vi "Noise (G3)-Create (Inverse Filtered).vi"(0 "Noise In":T6={"Properties"={"InvFilt"=TRUE, "Aweight"=FALSE, "Seed"=0, "Tokens"=0, "Brickwall"=FALSE}, "Data"={"TokenNum"=0}}, 5 "Level In":T4={"Level"=65.0, "Units"=enum."dB SPL", "Max"=129.40374449454038, "Data"={"Multiplier"=0.0, "Cal File"=path "C:/Data/Calibrations/InsertRight.calib", "Cal"={"Freq (Hz)"=array[999 elements], "Mag (dB SPL)"=array[999 elements], "Phase (deg)"=array[999 elements]}, "audiogram"=path "C:/Data/XYZ DATA/XYZ999/Right.txt"}}, 7 "Filter In":T1={"Type"=enum."Bandpass", "CF (kHz)"=3.0, "BW (kHz)"=1.0, "Cascade"=FALSE, "Quadrature"=FALSE, "Scale Factor"=0.618300269961, "Stages"=[{"IIR Filter"={"filter structure"=enum."IIR 4th Order", "Reverse Coefficients"=[-0.201940179927, 0.9304964170487, -0.1627584962201, 0.7169277799719, -0.188771055144, 0.7375967101194, -0.1003225284339, 0.3609942594263, -0.1818754527879, 0.63659078182, -0.06762987697315, 0.1746207484038, -0.1788768489915, 0.5926676052203, -0.05341323516015, 0.09357484569324], "Forward Coefficients"=[0.1997628457009, 0.0, -0.3995256914017, 0.0, 0.1997628457009, 0.1583503333203, 0.0, -0.3167006666407, 0.0, 0.1583503333203, 0.1366659600116, 0.0, -0.2733319200231, 0.0, 0.1366659600116, 0.1272363495488, 0.0, -0.2544726990976, 0.0, 0.1272363495488]}, "State"=[]}], "Class"=enum."Butterworth", "Order"=8, "BWUnits"=enum."Linear"} {"Stages"."IIR Filter"."Forward Coefficients" format="%.4f"; "Stages"."IIR Filter"."Reverse Coefficients" format="%.4f"}, 9 "Fs (Hz)":dbl=50000.0, 11 "error in (no error)":errorcluster, 12 "Token length (s)":dbl=7.146) -> (4 "Noise Out":T6={"Properties"={"InvFilt"=TRUE, "Aweight"=FALSE, "Seed"=0, "Tokens"=0, "Brickwall"=FALSE}, "Data"={"TokenNum"=0}}, 6 "Level Out":T4={"Level"=65.0, "Units"=enum."dB SPL", "Max"=129.02741664769067, "Data"={"Multiplier"=0.0, "Cal File"=path "C:/Data/Calibrations/InsertRight.calib", "Cal"={"Freq (Hz)"=array[999 elements], "Mag (dB SPL)"=array[999 elements], "Phase (deg)"=array[999 elements]}, "audiogram"=path "C:/Data/XYZ DATA/XYZ999/Right.txt"}}, 8 "Filter Out":T1={"Type"=enum."Bandpass", "CF (kHz)"=3.0, "BW (kHz)"=1.0, "Cascade"=FALSE, "Quadrature"=FALSE, "Scale Factor"=0.618300269961, "Stages"=[{"IIR Filter"={"filter structure"=enum."IIR 4th Order", "Reverse Coefficients"=[-0.201940179927, 0.9304964170487, -0.1627584962201, 0.7169277799719, -0.188771055144, 0.7375967101194, -0.1003225284339, 0.3609942594263, -0.1818754527879, 0.63659078182, -0.06762987697315, 0.1746207484038, -0.1788768489915, 0.5926676052203, -0.05341323516015, 0.09357484569324], "Forward Coefficients"=[0.1997628457009, 0.0, -0.3995256914017, 0.0, 0.1997628457009, 0.1583503333203, 0.0, -0.3167006666407, 0.0, 0.1583503333203, 0.1366659600116, 0.0, -0.2733319200231, 0.0, 0.1366659600116, 0.1272363495488, 0.0, -0.2544726990976, 0.0, 0.1272363495488]}, "State"=[]}], "Class"=enum."Butterworth", "Order"=8, "BWUnits"=enum."Linear"} {"Stages"."IIR Filter"."Forward Coefficients" format="%.4f"; "Stages"."IIR Filter"."Reverse Coefficients" format="%.4f"}, 10 "InvFilter Noise":dbl[](array[numeric]), 15 "error out":errorcluster)   [LabVIEW 2020]
uses:
  Noise (G3).ctl
  Noise (G3).Properties.ctl
  Noise (G3).Data.ctl
  XControls/Level (G3)/Level Data.ctl
  XControls/Level (G3)/Level Units (G3).ctl
  XControls/Filter (G3)/Filter Data.ctl
  XControls/Filter (G3)/Filter Type.ctl
  Filter VIs/Filter-Bandwidth Units.ctl
  Calibration VIs/Inverse Filter VIs/InvFilt-Params.ctl
  XControls/Filter (G3)/Filter (G3).xctl
  XControls/Level (G3)/Level (G3).xctl
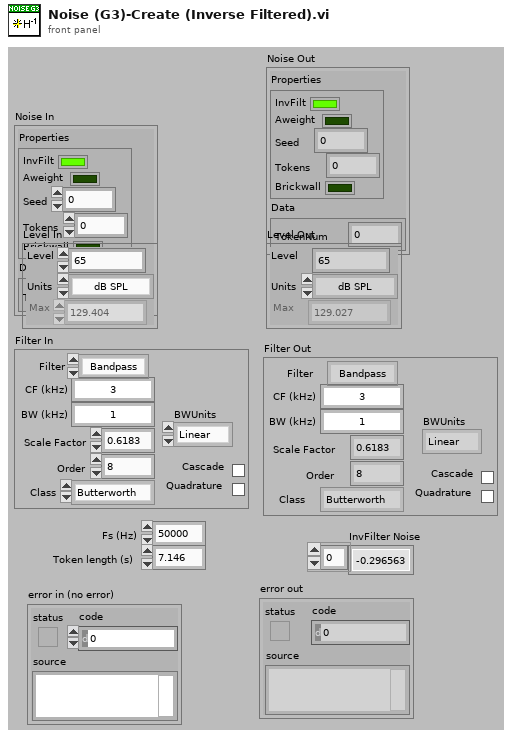
[diagram p1: front panel]
types:
  T1 = typedef "Filter (G3).xctl/Filter Data.ctl" = cluster{"Type":T2, "CF (kHz)":dbl, "BW (kHz)":dbl, "Cascade":bool, "Quadrature":bool, "Scale Factor":dbl, "Stages":cluster{"IIR Filter":cluster{"filter structure":enum32{"IIR 2nd Order", "IIR 4th Order"}, "Reverse Coefficients":dbl[], "Forward Coefficients":dbl[]}, "State":dbl[]}[], "Class":enum16{"Elliptic", "Butterworth"}, "Order":i32, "BWUnits":T3}
  T2 = typedef "Filter (G3).xctl/Filter Type.ctl" = enum16{"OFF", "Lowpass", "Highpass", "Bandpass", "Bandstop"}
  T3 = typedef "Filter-Bandwidth Units.ctl" = enum16{"Linear", "Octaves", "Min-Max"}
  T4 = typedef "Level (G3).xctl/Level Data.ctl" = cluster{"Level":dbl, "Units":T5, "Max":dbl, "Data":cluster{"Multiplier":dbl, "Cal File":path, "Cal":cluster{"Freq (Hz)":dbl[], "Mag (dB SPL)":dbl[], "Phase (deg)":dbl[]}, "audiogram":path}}
  T5 = typedef "Level (G3).xctl/Level Units (G3).ctl" = enum16{"dB atten", "dB SPL", "dB re 1 Vrms", "dB V/Hz½", "mW", "dB HL", "Volts", "dB mW"}
  T6 = typedef "Noise (G3).ctl" = cluster{"Properties":T7, "Data":T8}
  T7 = typedef "Noise (G3).Properties.ctl" = cluster{"InvFilt":bool, "Aweight":bool, "Seed":i32, "Tokens":i32, "Brickwall":bool}
  T8 = typedef "Noise (G3).Data.ctl" = cluster{"TokenNum":i32}
  T9 = typedef "InvFilt-Params.ctl" = cluster{"Min Frequency (Hz)":dbl, "Max Frequency (Hz)":dbl, "Length (points)":i32, "Sampling rate (Hz)":dbl, "Delay (ms)":dbl, "Linear phase":bool}
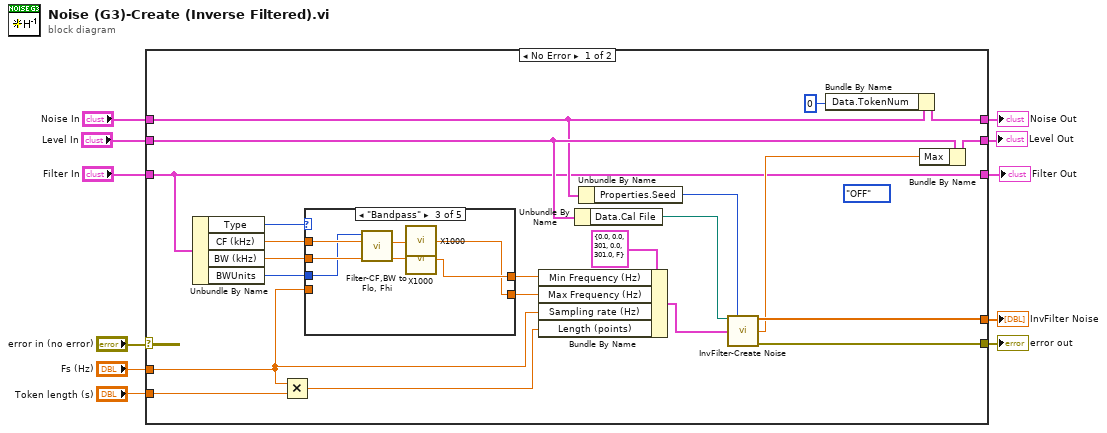
[diagram p0: block diagram]
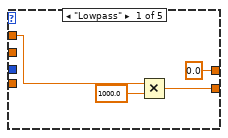
[diagram p2: hidden frame]
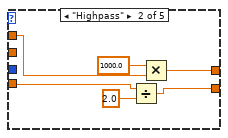
[diagram p3: hidden frame]
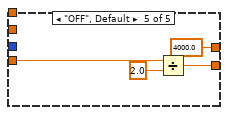
[diagram p5: hidden frame]
diagram:
  n1 = case shown="No Error" "error in (no error)" {
    selector: "error in (no error)" -> [_ w58]
    tunnel: [w21 w58] -> w10
    tunnel: "Noise In" -> [w15 w57]
    tunnel: "Fs (Hz)" -> [w24 _]
    tunnel: "Token length (s)" -> [w26 _]
    tunnel: [w23 w57] -> w4
    tunnel: [w20 _] -> w7
    tunnel: "Filter In" -> [w13 w55]
    tunnel: "Level In" -> [w18 w56]
    tunnel: [w17 w56] -> w2
    tunnel: [w13 w55] -> w1
    frame No Error {
      (unwired) Filter_Type."OFF" ("Type")
      n2 = Unbundle By Name(w13) -> ("Type"=w31:T2, "CF (kHz)"=w28:dbl, "BW (kHz)"=w27:dbl, "BWUnits"=w12:T3)
      n3 = Multiply(x=w24, y=w26) -> (x*y=w25:dbl)
      n4 = case shown="\"Bandpass\"" w31 {
        tunnel: [0.0 w39 w45 _ 4000.0] -> w30
        tunnel: [w35 w41 w44 _ w53] -> w29
        tunnel: w24 -> [_ w42 _ _ w52]
        tunnel: w28 -> [w36 w40 w48 _ _]
        tunnel: w27 -> [_ _ w47 _ _]
        tunnel: w12 -> [_ _ w46 _ _]
        frame "Lowpass" {
          n5 = Multiply(x=w36, y=1000.0) -> (x*y=w35:dbl)
        }
        frame "Highpass" {
          n6 = Divide(x=w42, y=2.0) -> (x/y=w41:dbl)
          n7 = Multiply(x=1000.0, y=w40) -> (x*y=w39:dbl)
        }
        frame "Bandpass" {
          n8 = call "Filter-CF,BW to Flo, Fhi.vi"("BW"=w47, "CF (kHz)"=w48, "BWUnits"=w46) -> ("Fmin"=w50:dbl, "Fmax"=w49:dbl)  [unwired: 7 in]
          n9 = call "X1000.vi"("X"=w49) -> ("X/1000"=w44:dbl)
          n10 = call "X1000.vi"("X"=w50) -> ("X/1000"=w45:dbl)
        }
        frame "Bandstop" {
        }
        frame "OFF", Default {
          n11 = Divide(x=w52, y=2.0) -> (x/y=w53:dbl)
        }
      }
      n12 = Bundle By Name(cluster=T9 {"Min Frequency (Hz)"=0.0, "Max Frequency (Hz)"=0.0, "Length (points)"=301, "Sampling rate (Hz)"=0.0, "Delay (ms)"=301.0, "Linear phase"=FALSE} ("InvFilt Params"), "Min Frequency (Hz)"=w30, "Max Frequency (Hz)"=w29, "Sampling rate (Hz)"=w24, "Length (points)"=w25) -> (w33:T9)
      n13 = Unbundle By Name(w18) -> ("Data.Cal File"=w19:path)
      n14 = Unbundle By Name(w15) -> ("Properties.Seed"=w14:i32)
      n15 = call "InvFilter-Create Noise.vi"("Calibration File"=w19, "seed"=w14, "InvFilt Params"=w33) -> ("InvFilter Noise"=w20:dbl[], "Max Level"=w16:dbl, "error out"=w21:errorcluster)  [unwired: 9 in, 1 out]
      n16 = Bundle By Name(cluster=w15, "Data.TokenNum"=0 ("Waveform.Noise.CurPt")) -> (w23:T6)
      n17 = Bundle By Name(cluster=w18, "Max"=w16) -> (w17:T4)
    }
    frame Error {
    }
  }
  "error out" <- w10
  "InvFilter Noise" <- w7
  "Noise Out" <- w4
  "Level Out" <- w2
  "Filter Out" <- w1
